vi "Set IO Capabilities.vi"(8 "error in":errorcluster, 10 "Capabilities":T1, 11 "CiA401 Generic IO Profile in":refnum<class "CiA401 Generic IO Profile.lvclass">) -> (0 "error out":errorcluster, 3 "CiA401 Generic IO Profile out":refnum<class "CiA401 Generic IO Profile.lvclass">)   [LabVIEW 2020, in "CiA401 Generic IO Profile.lvclass"]
uses:
  CiA401 Generic IO Profile.lvclass
  CiA401 Generic IO Profile.lvclass/CiA401 Generic IO Profile.ctl
  IO Capabilities.ctl
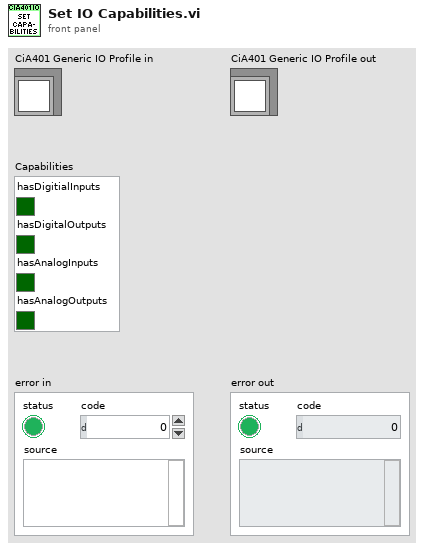
[diagram p1: front panel]
types:
  T1 = typedef "CiA401 Generic IO Profile.lvclass/IO Capabilities.ctl" = cluster{"hasDigitialInputs":bool, "hasDigitalOutputs":bool, "hasAnalogInputs":bool, "hasAnalogOutputs":bool}
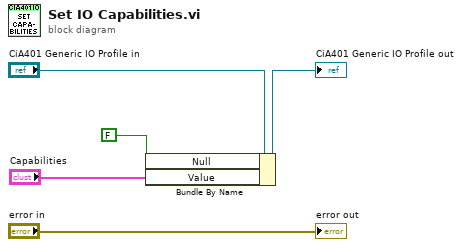
[diagram p0: block diagram]
diagram:
  n1 = Bundle By Name(cluster="CiA401 Generic IO Profile in", "Null"=FALSE ("Capabilities.Null"), "Value"="Capabilities") -> (→"CiA401 Generic IO Profile out":refnum<class "CiA401 Generic IO Profile.lvclass">)
  "error out" <- "error in"
